vi "BasicAnalysis.vi"(9 "Units":enum16{"True RMS", "Noise RMS"}(ring), 11 "Data (Volts)":dbl[][](array[numeric])) -> (1 "Analysis Data":string[][](array[string]), 2 "Row Headers":string[](array[string]), 3 "Column Headers":string[](array[string]))   [LabVIEW 2010]
uses:
  <vilib>/Analysis/5stat.llb/RMS (DBL).vi
  <vilib>/Analysis/NI_AALBase.lvlib
  <vilib>/Analysis/NI_AALPro.lvlib
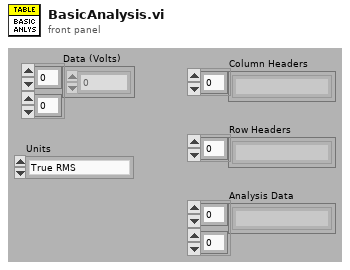
[diagram p1: front panel]
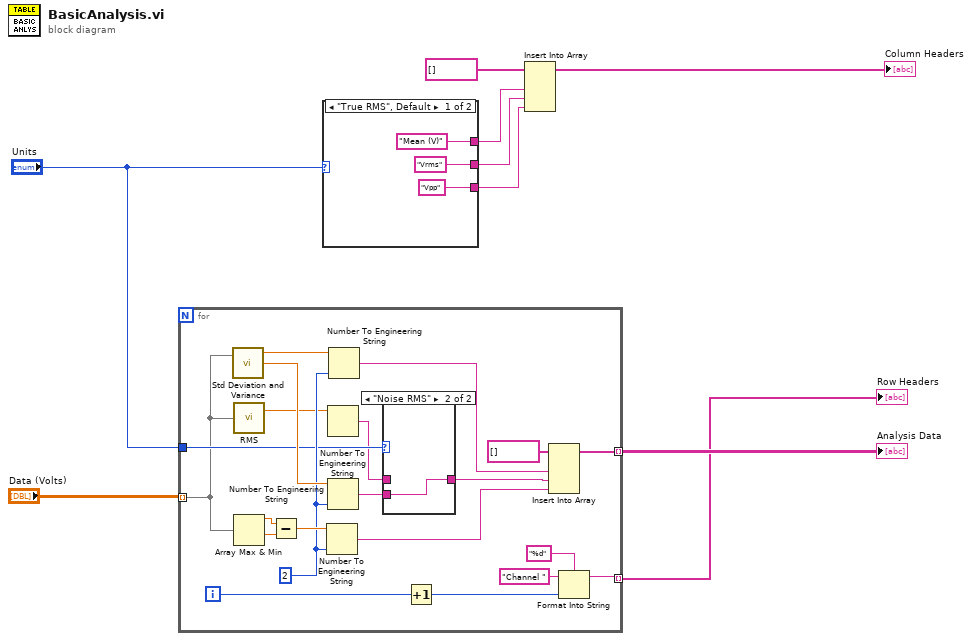
[diagram p0: block diagram]
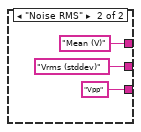
[diagram p2: hidden frame]
diagram:
  n1 = for {
    tunnel: "Data (Volts)" -> [w12] mode=indexing
    tunnel: [w16] -> w9 mode=indexing
    tunnel: [w22] -> w8 mode=indexing
    tunnel: "Units" -> [w14]
    i -> [w25]
    w20 = i16 2 ("precision (6)")
    n2 = call <vilib>:"Std Deviation and Variance.vi"("X"=w12) -> ("mean"=w30:dbl, "standard deviation"=w27:dbl)  [unwired: 1 in, 1 out]
    n3 = call-poly <vilib>:"RMS.vi"("X"=w12) -> ("rms value"=w11:dbl)  [unwired: 1 out]
    n4 = Array Max & Min(array=w12) -> (max value=w29:dbl, min value=w28:dbl)  [unwired: 2 out]
    n5 = Subtract(x=w29, y=w28) -> (x-y=w26:dbl)
    n6 = Number To Engineering String(2:w20, 4:w26) -> (0:w17:string)  [unwired: 2 out]
    n7 = Number To Engineering String(4:w11) -> (0:w10:string)  [unwired: 3 out]
    n8 = Number To Engineering String(2:w20, 4:w27) -> (0:w15:string)  [unwired: 2 out]
    n9 = Number To Engineering String(2:w20, 4:w30) -> (0:w18:string)  [unwired: 2 out]
    n10 = case shown="\"Noise RMS\"" w14 {
      tunnel: w15 -> [_ w32]
      tunnel: [w31 w32] -> w13
      tunnel: w10 -> [w31 _]
      frame "True RMS", Default {
      }
      frame "Noise RMS" {
      }
    }
    n11 = Increment(x=w25) -> (x+1=w21:i32)
    n12 = Insert Into Array(array=string[] [], new element #1=w18, new element #2=w13, new element #3=w17) -> (w16:string[])  [unwired: 1 in]
    n13 = Format Into String(format string="%d", initial string="Channel ", w21) -> (resulting string=w22:string)  [unwired: 1 in, 1 out]
  }
  "Analysis Data" <- w9
  "Row Headers" <- w8
  n14 = case shown="\"True RMS\", Default" "Units" {
    tunnel: ["Vrms" ("element") "Vrms (stddev)" ("element")] -> w4
    tunnel: ["Mean (V)" ("element") "Mean (V)" ("element")] -> w3
    tunnel: ["Vpp" ("element") "Vpp" ("element")] -> w5
    frame "True RMS", Default {
    }
    frame "Noise RMS" {
    }
  }
  n15 = Insert Into Array(array=string[] [], new element #1=w3, new element #2=w4, new element #3=w5) -> (→"Column Headers":string[])  [unwired: 1 in]
